vi "Script Cases.vi"(0 "Primitives & Arguments":T1) -> ()   [LabVIEW 2014]
uses:
  Begin/Global Variables.vi
  <vilib>/Utility/file.llb/Write To Spreadsheet File (string).vi
  Begin/Global RefNums.vi
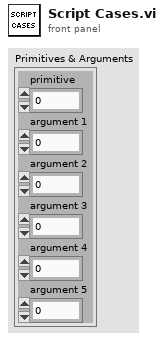
[diagram p1: front panel]
types:
  T1 = cluster{"primitive":i32, "argument 1":dbl, "argument 2":dbl, "argument 3":dbl, "argument 4":dbl, "argument 5":dbl}
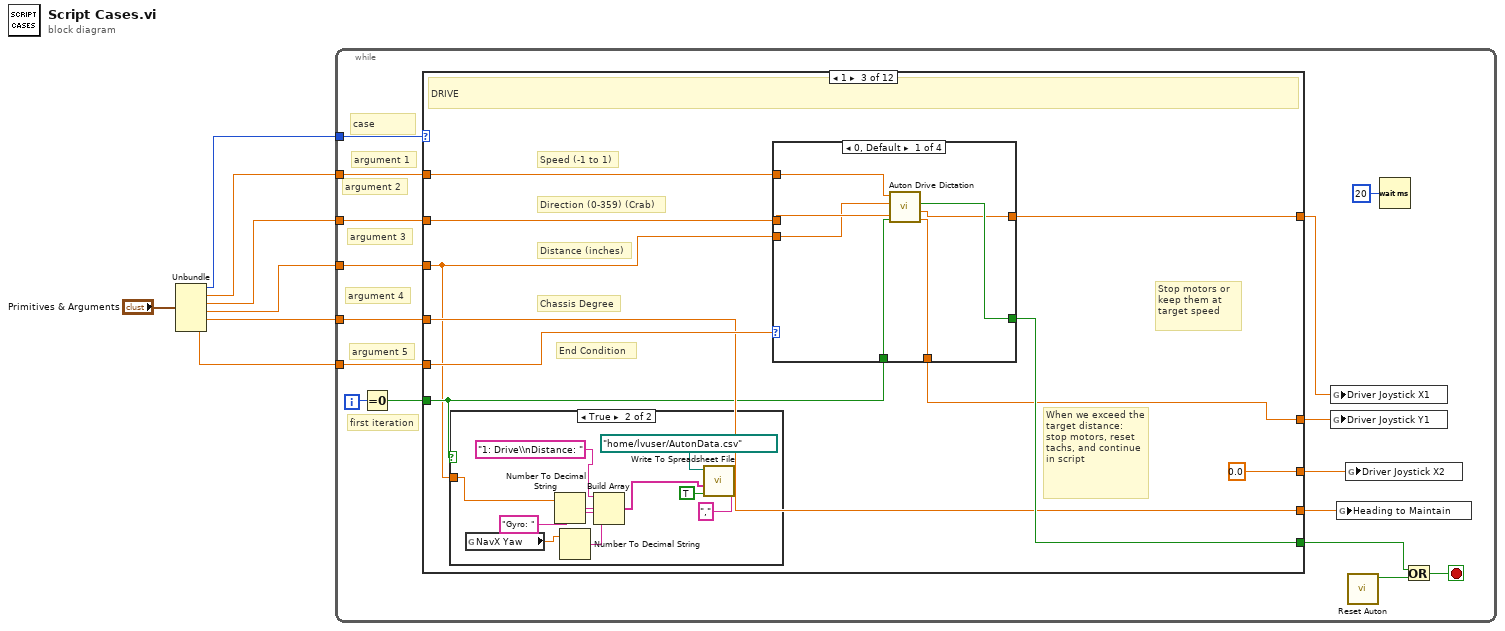
[diagram p0: block diagram]
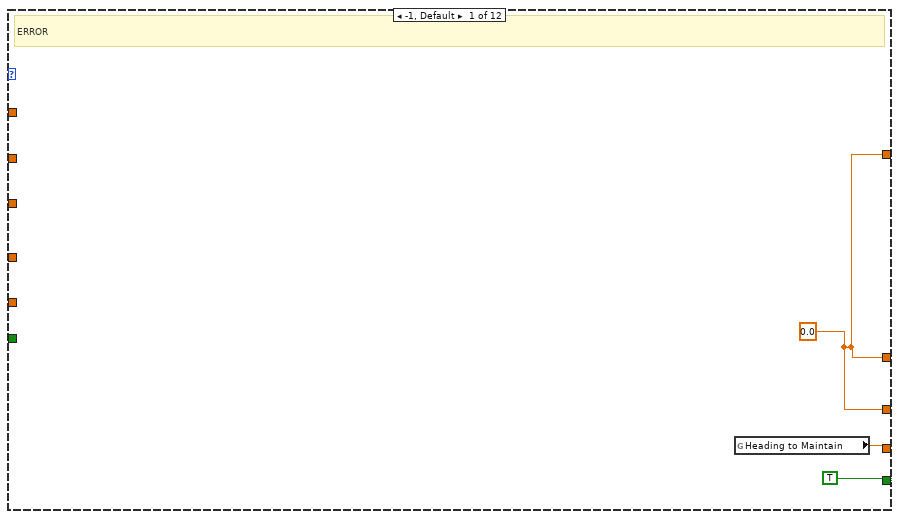
[diagram p2: hidden frame]
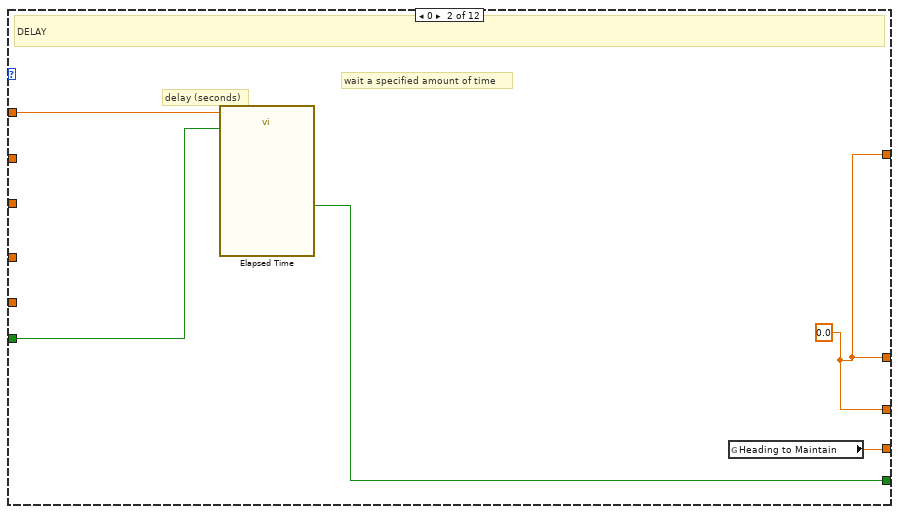
[diagram p3: hidden frame]
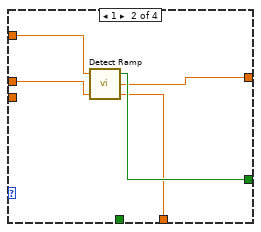
[diagram p5: hidden frame]
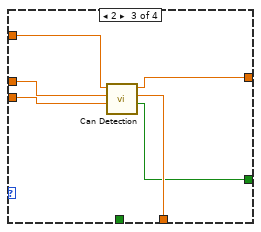
[diagram p6: hidden frame]
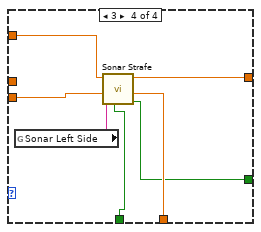
[diagram p7: hidden frame]
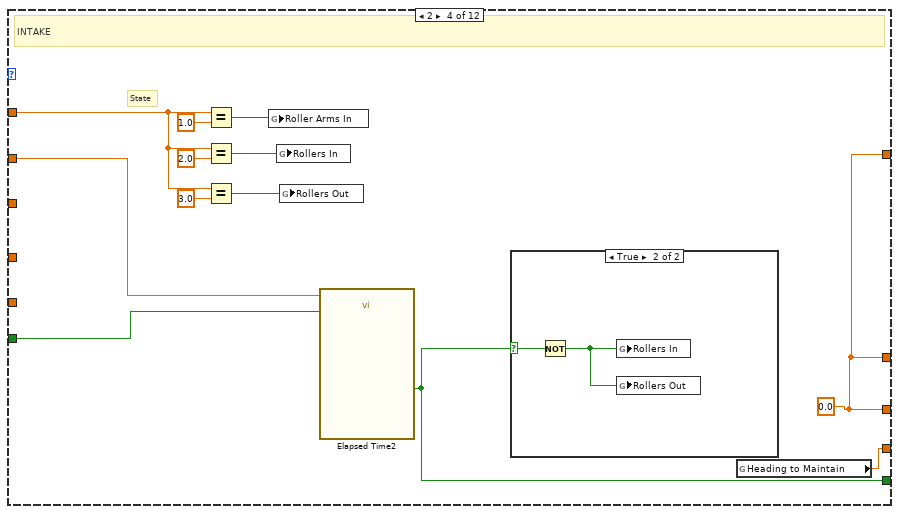
[diagram p8: hidden frame]
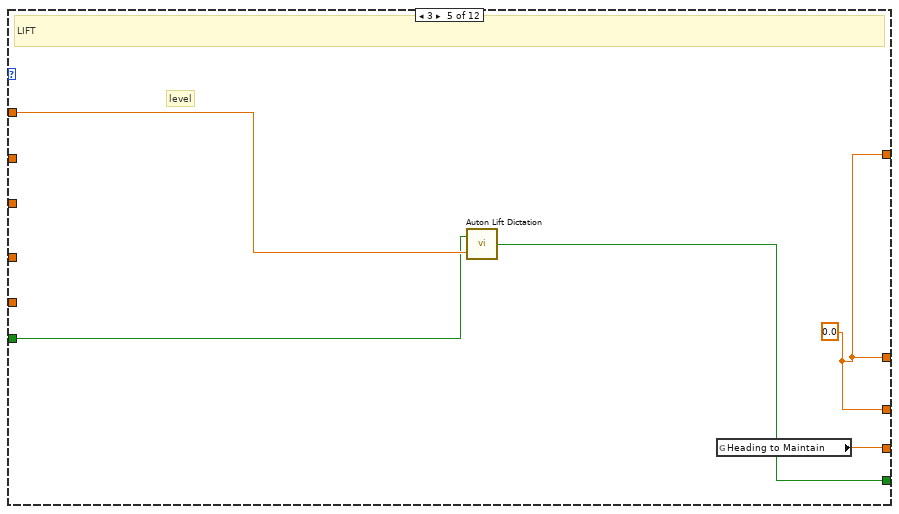
[diagram p10: hidden frame]
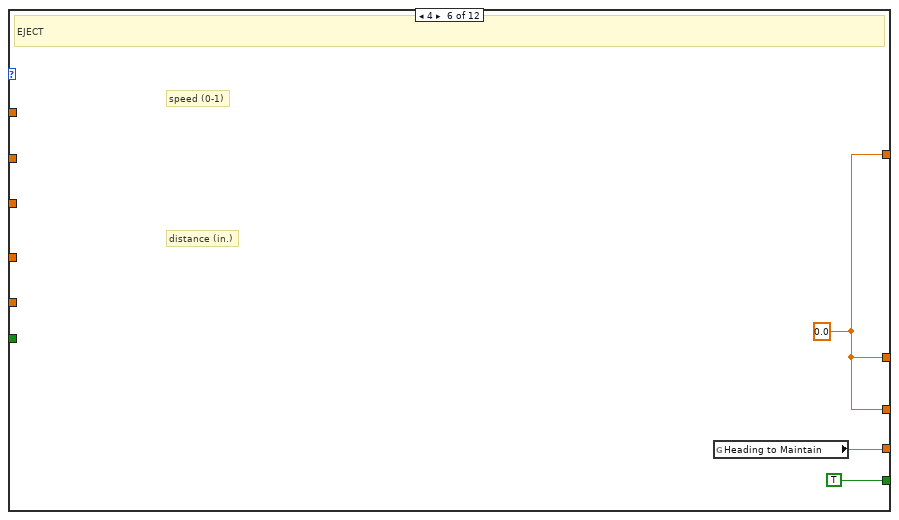
[diagram p11: hidden frame]
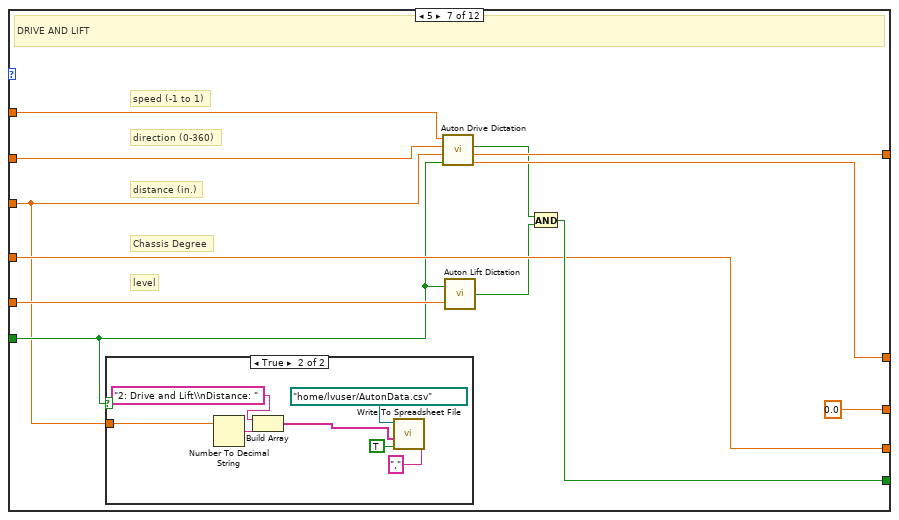
[diagram p12: hidden frame]
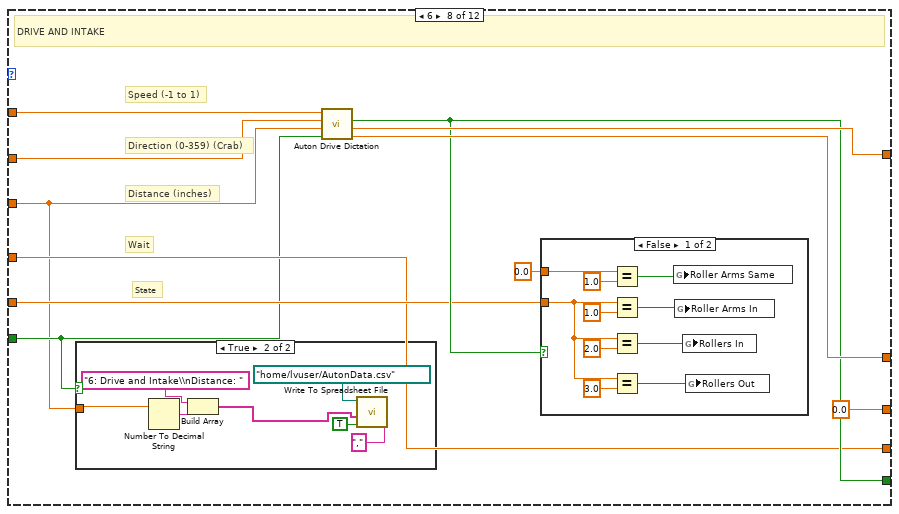
[diagram p14: hidden frame]
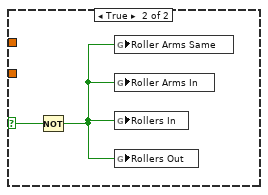
[diagram p16: hidden frame]
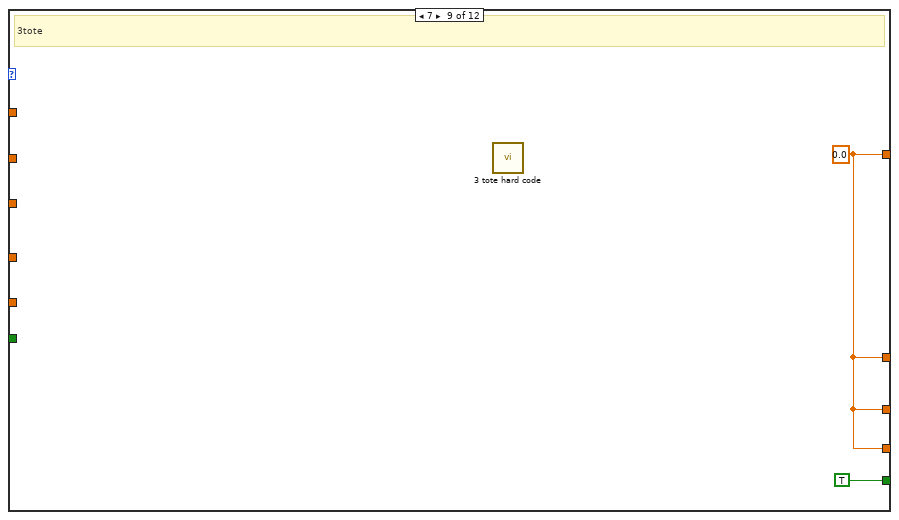
[diagram p17: hidden frame]
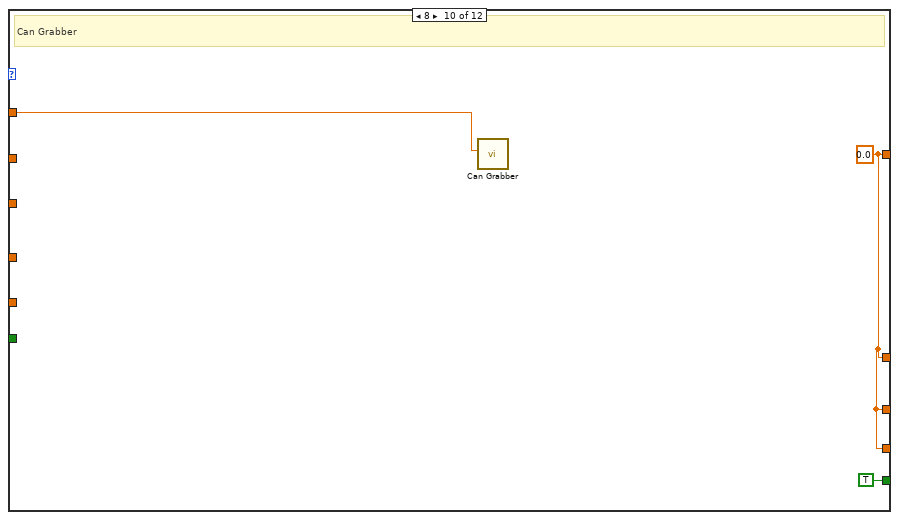
[diagram p18: hidden frame]
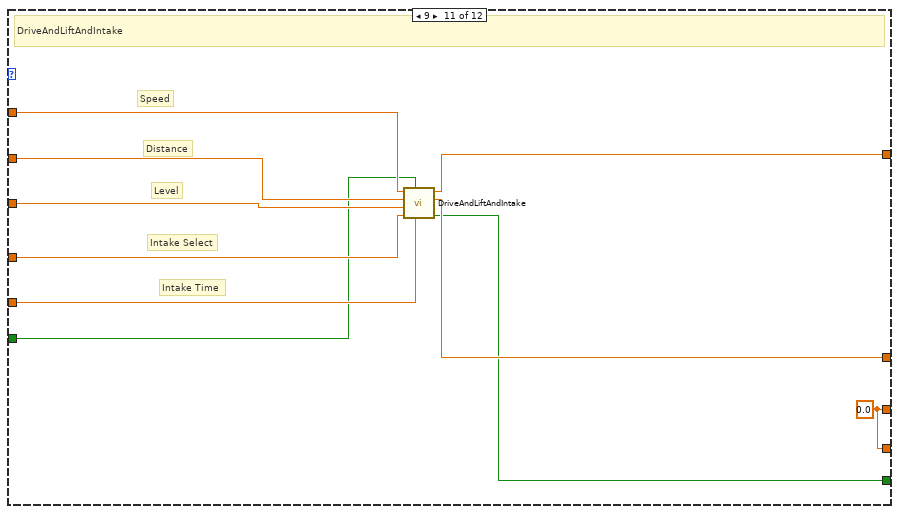
[diagram p19: hidden frame]
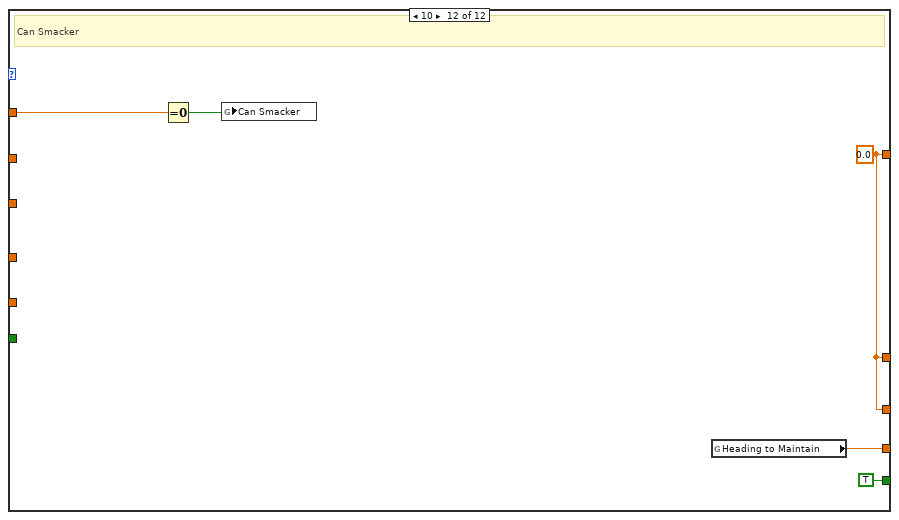
[diagram p20: hidden frame]
diagram:
  n1 = Unbundle("Primitives & Arguments") -> ("primitive"=w6:i32, "argument 1"=w5:dbl, "argument 2"=w4:dbl, "argument 3"=w3:dbl, "argument 4"=w2:dbl, "argument 5"=w1:dbl)
  n2 = while {
    tunnel: w5 -> [w23]
    tunnel: w4 -> [w22]
    tunnel: w3 -> [w21]
    tunnel: w2 -> [w20]
    tunnel: w1 -> [w19]
    tunnel: w6 -> [w18]
    i -> [w17]
    stop <- w9 stop-if-true
    # "first iteration"
    # "case"
    # "argument 5"
    # "argument 4"
    # "argument 3"
    # "argument 2"
    # "argument 1"
    n3 = Equal To 0?(x=w17) -> (x = 0?=w16:bool)
    n4 = case shown="1" w18 {
      tunnel: w23 -> [_ w31 w40 w85 w95 _ w109 w128 _ w150 w162 w167]
      tunnel: w22 -> [_ _ w39 w81 _ _ w108 w127 _ _ w161 _]
      tunnel: w21 -> [_ _ w32 _ _ _ w101 w118 _ _ w160 _]
      tunnel: w20 -> [_ _ w36 _ _ _ w103 w120 _ _ w158 _]
      tunnel: w19 -> [_ _ w37 _ _ _ w107 w122 _ _ w159 _]
      tunnel: [TRUE w29 w38 w80 w94 TRUE w106 w124 TRUE ("Distance Reached?") TRUE ("Distance Reached?") w155 TRUE ("Done?")] -> w10
      tunnel: w16 -> [_ w30 w33 w79 w92 _ w102 w119 _ _ w153 _]
      tunnel: [w25 w28 0.0 ("argument 1") w78 w93 w97 0.0 ("argument 1") 0.0 ("argument 1") w148 w152 w154 w165] -> w15
      tunnel: [w24 w27 w36 w77 w91 w96 w103 w120 w148 w152 w154 w164] -> w14
      tunnel: [w25 w28 w35 w78 w93 w97 w105 w126 w148 w152 w157 w165] -> w12
      tunnel: [w25 w28 w34 w78 w93 w97 w104 w125 w148 w152 w156 w165] -> w11
      frame -1, Default {
        w25 = 0.0 ("argument 1")
        # "ERROR"
        n5 = global read "Global Variables.vi" "Heading to Maintain"() -> (w24:dbl)
      }
      frame 0 {
        w28 = 0.0 ("argument 1")
        # "wait a specified amount of time"
        # "delay (seconds)"
        # "DELAY"
        n6 = call "Elapsed Time"("Time Target (s)"=w31, "Reset"=w30) -> ("Time has Elapsed"=w29:bool)  [unwired: 10 in, 7 out]
        n7 = global read "Global Variables.vi" "Heading to Maintain"() -> (w27:dbl)
      }
      frame 1 {
        # "Chassis Degree"
        # "End Condition"
        # "When we exceed the target distance: stop motors, reset tachs, and continue in script"
        # "Stop motors or keep them at target speed"
        # "Distance (inches)"
        # "Direction (0-359) (Crab)"
        # "Speed (-1 to 1)"
        # "DRIVE"
        n8 = case shown="True" w33 {
          tunnel: w32 -> [_ w46]
          frame False {
          }
          frame True {
            n9 = global read "Global Variables.vi" "NavX Yaw"() -> (w47:dbl)
            n10 = Number To Decimal String(number=w46) -> (decimal integer string=w48:string)  [unwired: 1 in]
            n11 = Number To Decimal String(number=w47) -> (decimal integer string=w43:string)  [unwired: 1 in]
            n12 = Build Array("1: Drive\\nDistance: " ("text"), w48, "Gyro: " ("element"), w43) -> (w42:string[])
            n13 = call-poly <vilib>:"Write To Spreadsheet File.vi"("delimiter (\\t)"="," ("delimiter (\\t)"), "append to file? (new file:F)"=TRUE, "1D data"=w42, "file path (dialog if empty)"=path "/home/lvuser/AutonData.csv" ("file path (use dialog)")) -> ()  [unwired: 4 in, 1 out]
          }
        }
        n14 = case shown="0, Default" w37 {
          tunnel: w40 -> [w58 w63 w67 w70]
          tunnel: w39 -> [w57 w62 w66 _]
          tunnel: w32 -> [w56 _ w65 w76]
          tunnel: [w55 w61 w64 w73] -> w38
          tunnel: w33 -> [w54 _ _ w71]
          tunnel: [w53 w60 w69 w75] -> w35
          tunnel: [w52 w59 w68 w74] -> w34
          frame 0, Default {
            n15 = call "Auton Drive Dictation.vi"("Reset Encoders"=w54, "Distance (inches)"=w56, "Direction (0-359)"=w57, "Speed (-1 to 1)"=w58) -> ("Joy Y"=w52:dbl, "Joy X"=w53:dbl, "Distance Reached?"=w55:bool)  [unwired: 5 in]
          }
          frame 1 {
            n16 = call "Detect Ramp.vi"("Direction"=w62, "Speed"=w63) -> ("JoyY"=w59:dbl, "Joy X"=w60:dbl, "Finished"=w61:bool)  [unwired: 1 in]
          }
          frame 2 {
            n17 = call "Can Detection.vi"("Stop Voltage"=w65, "Direction (0-359)"=w66, "Speed"=w67) -> ("Distance Reached?"=w64:bool, "Joy Y"=w68:dbl, "Joy X"=w69:dbl)  [unwired: 6 in]
          }
          frame 3 {
            n18 = global read "Global RefNums.vi" "Sonar Left Side"() -> (w72:string)
            n19 = call "Sonar Strafe.vi"("reinitialize? (F)"=w71, "Sonar Side"=w72, "Desired Wall Distance"=w76, "Speed"=w70) -> ("Distance Reached?"=w73:bool, "Joy Y"=w74:dbl, "Joy X"=w75:dbl)  [unwired: 5 in]
          }
        }
      }
      frame 2 {
        w78 = 0.0 ("argument 1")
        # "State"
        # "INTAKE"
        n20 = Equal?(x=w85, y=1.0) -> (x = y?=w82:bool)
        n21 = Equal?(x=w85, y=2.0) -> (x = y?=w83:bool)
        n22 = Equal?(x=w85, y=3.0) -> (x = y?=w84:bool)
        n23 = global write "Global Variables.vi" "Roller Arms In"(w82) -> ()
        n24 = global write "Global Variables.vi" "Rollers In"(w83) -> ()
        n25 = global write "Global Variables.vi" "Rollers Out"(w84) -> ()
        n26 = call "Elapsed Time2"("Time Target (s)"=w81, "Reset"=w79) -> ("Time has Elapsed"=w80:bool)  [unwired: 10 in, 7 out]
        n27 = case shown="True" w80 {
          selector: w80 -> [_ w90]
          frame False {
          }
          frame True {
            n28 = Not(x=w90) -> (.not. x?=w89:bool)
            n29 = global write "Global Variables.vi" "Rollers In"(w89) -> ()
            n30 = global write "Global Variables.vi" "Rollers Out"(w89) -> ()
          }
        }
        n31 = global read "Global Variables.vi" "Heading to Maintain"() -> (w77:dbl)
      }
      frame 3 {
        w93 = 0.0 ("argument 1")
        # "level"
        # "LIFT"
        n32 = call "Auton Lift Dictation.vi"("Level"=w95, "First Iteration"=w92) -> ("Lift Sequence Done"=w94:bool)
        n33 = global read "Global Variables.vi" "Heading to Maintain"() -> (w91:dbl)
      }
      frame 4 {
        w97 = 0.0 ("argument 1")
        # "distance (in.)"
        # "speed (0-1)"
        # "EJECT"
        n34 = global read "Global Variables.vi" "Heading to Maintain"() -> (w96:dbl)
      }
      frame 5 {
        # "Chassis Degree"
        # "level"
        # "distance (in.)"
        # "direction (0-360)"
        # "speed (-1 to 1)"
        # "DRIVE AND LIFT"
        n35 = case shown="True" w102 {
          tunnel: w101 -> [_ w117]
          frame False {
          }
          frame True {
            n36 = Number To Decimal String(number=w117) -> (decimal integer string=w112:string)  [unwired: 1 in]
            n37 = Build Array("2: Drive and Lift\\nDistance: " ("text"), w112) -> (w111:string[])
            n38 = call-poly <vilib>:"Write To Spreadsheet File.vi"("delimiter (\\t)"="," ("delimiter (\\t)"), "append to file? (new file:F)"=TRUE, "1D data"=w111, "file path (dialog if empty)"=path "/home/lvuser/AutonData.csv" ("file path (use dialog)")) -> ()  [unwired: 4 in, 1 out]
          }
        }
        n39 = call "Auton Drive Dictation.vi"("Reset Encoders"=w102, "Distance (inches)"=w101, "Direction (0-359)"=w108, "Speed (-1 to 1)"=w109) -> ("Joy Y"=w104:dbl, "Joy X"=w105:dbl, "Distance Reached?"=w100:bool)  [unwired: 5 in]
        n40 = call "Auton Lift Dictation.vi"("Level"=w107, "First Iteration"=w102) -> ("Lift Sequence Done"=w99:bool)
        n41 = And(x=w100, y=w99) -> (x .and. y?=w106:bool)
      }
      frame 6 {
        # "State"
        # "Wait"
        # "Distance (inches)"
        # "Direction (0-359) (Crab)"
        # "Speed (-1 to 1)"
        # "DRIVE AND INTAKE"
        n42 = case shown="True" w119 {
          tunnel: w118 -> [_ w130]
          frame False {
          }
          frame True {
            n43 = Number To Decimal String(number=w130) -> (decimal integer string=w132:string)  [unwired: 1 in]
            n44 = Build Array("6: Drive and Intake\\nDistance: " ("text"), w132) -> (w129:string[])
            n45 = call-poly <vilib>:"Write To Spreadsheet File.vi"("delimiter (\\t)"="," ("delimiter (\\t)"), "append to file? (new file:F)"=TRUE, "1D data"=w129, "file path (dialog if empty)"=path "/home/lvuser/AutonData.csv" ("file path (use dialog)")) -> ()  [unwired: 4 in, 1 out]
          }
        }
        n46 = call "Auton Drive Dictation.vi"("Reset Encoders"=w119, "Distance (inches)"=w118, "Direction (0-359)"=w127, "Speed (-1 to 1)"=w128) -> ("Joy Y"=w125:dbl, "Joy X"=w126:dbl, "Distance Reached?"=w124:bool)  [unwired: 5 in]
        n47 = case shown="False" w124 {
          selector: w124 -> [_ w147]
          tunnel: w122 -> [w139 _]
          tunnel: 0.0 ("argument 4") -> [w136 _]
          frame False {
            n48 = Equal?(x=w136, y=1.0) -> (x = y?=w137:bool)
            n49 = Equal?(x=w139, y=1.0) -> (x = y?=w145:bool)
            n50 = Equal?(x=w139, y=2.0) -> (x = y?=w144:bool)
            n51 = Equal?(x=w139, y=3.0) -> (x = y?=w143:bool)
            n52 = global write "Global Variables.vi" "Roller Arms Same"(w137) -> ()
            n53 = global write "Global Variables.vi" "Roller Arms In"(w145) -> ()
            n54 = global write "Global Variables.vi" "Rollers In"(w144) -> ()
            n55 = global write "Global Variables.vi" "Rollers Out"(w143) -> ()
          }
          frame True {
            n56 = Not(x=w147) -> (.not. x?=w146:bool)
            n57 = global write "Global Variables.vi" "Roller Arms Same"(w146) -> ()
            n58 = global write "Global Variables.vi" "Roller Arms In"(w146) -> ()
            n59 = global write "Global Variables.vi" "Rollers In"(w146) -> ()
            n60 = global write "Global Variables.vi" "Rollers Out"(w146) -> ()
          }
        }
      }
      frame 7 {
        w148 = 0.0 ("Joy X")
        # "3tote"
        n61 = call "3 tote hard code.vi"() -> ()  [unwired: 12 in]
      }
      frame 8 {
        w152 = 0.0 ("Joy X")
        # "Can Grabber"
        n62 = call "Can Grabber.vi"("Grabber State"=w150) -> ()  [unwired: 11 in]
      }
      frame 9 {
        w154 = 0.0 ("Joy X")
        # "Intake Time"
        # "Intake Select"
        # "Level"
        # "Distance"
        # "Speed"
        # "DriveAndLiftAndIntake"
        n63 = call "DriveAndLiftAndIntake.vi"("Intake Time"=w159, "First Iteration"=w153, "Intake Select"=w158, "Level"=w160, "Distance"=w161, "Speed"=w162) -> ("Done?"=w155:bool, "Joy Y"=w156:dbl, "Joy X"=w157:dbl)  [unwired: 3 in]
      }
      frame 10 {
        w165 = 0.0 ("Joy X")
        # "Can Smacker"
        n64 = Equal To 0?(x=w167) -> (x = 0?=w166:bool)
        n65 = global write "Global Variables.vi" "Can Smacker"(w166) -> ()
        n66 = global read "Global Variables.vi" "Heading to Maintain"() -> (w164:dbl)
      }
    }
    n67 = global write "Global Variables.vi" "Driver Joystick X1"(w12) -> ()
    n68 = global write "Global Variables.vi" "Driver Joystick Y1"(w11) -> ()
    n69 = global write "Global Variables.vi" "Heading to Maintain"(w14) -> ()
    n70 = global write "Global Variables.vi" "Driver Joystick X2"(w15) -> ()
    n71 = call "Reset Auton.vi"() -> ("Reset Auton"=w8:bool)  [unwired: 11 in]
    n72 = Wait (ms)(milliseconds to wait=u32 20) -> ()  [unwired: 1 out]
    n73 = Or(x=w10, y=w8) -> (x .or. y?=w9:bool)
  }
